vi "example.vi"() -> ()   [LabVIEW 2016]
uses:
  LS-H600-TCP Client.lvclass
  C:/Program Files (x86)/National Instruments/LabVIEW 2016/vi.lib/ActorFramework/Actor/Actor.lvclass
  LS-H600-TCP Client.lvclass/LS-H600-TCP Client.ctl
  <vilib>/ActorFramework/Message Enqueuer/Message Enqueuer.lvclass/Message Enqueuer.ctl
  <vilib>/ActorFramework/Message Enqueuer/Enqueue.vi
  C:/Program Files (x86)/National Instruments/LabVIEW 2016/vi.lib/ActorFramework/Message/Message.lvclass
  <vilib>/ActorFramework/Stop Msg/Stop Msg.lvclass
  <vilib>/ActorFramework/Message Priority Queue/Priority Enqueue.vi
  <vilib>/ActorFramework/Actor/Actor.lvclass
panel:
  out "连接错误":errorcluster
  out "数据输出":string
  out "data":T1
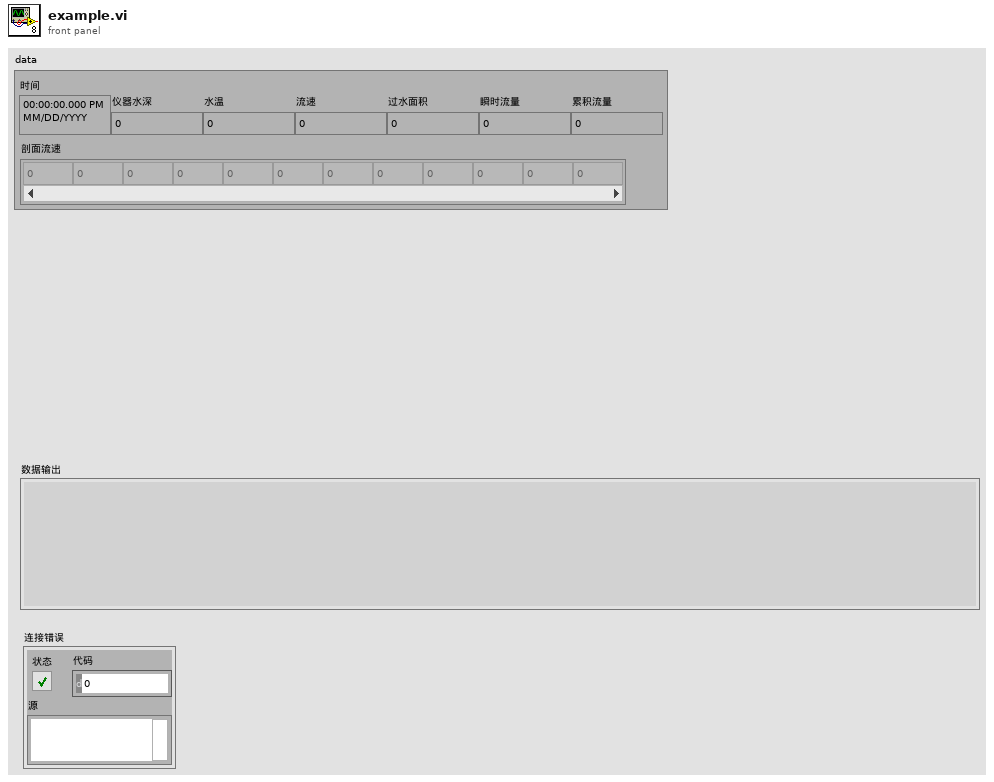
[diagram p1: front panel]
types:
  T1 = cluster{"时间":timestamp, "仪器水深":dbl, "水温":dbl, "流速":dbl, "过水面积":dbl, "瞬时流量":dbl, "累积流量":dbl, "剖面流速":dbl[]}
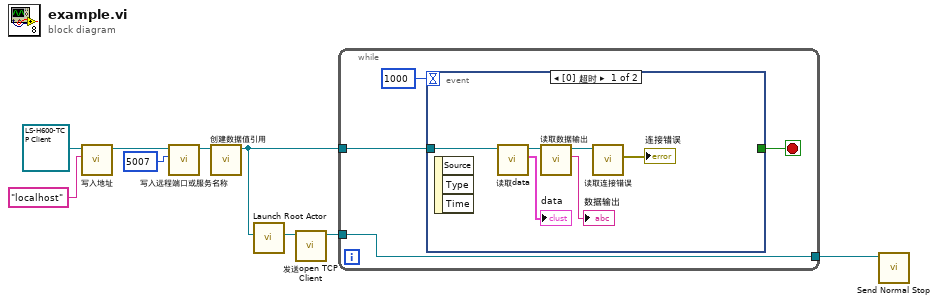
[diagram p0: block diagram]
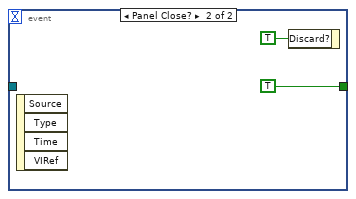
[diagram p2: hidden frame]
diagram:
  n1 = call "写入地址.vi"("地址"="localhost", "LS-H600-TCP Client输入"=refnum<class "LS-H600-TCP Client.lvclass"> refnum ("LS-H600-TCP Client.lvlib:LS-H600-TCP Client.lvclass")) -> ("LS-H600-TCP Client输出"=w8:refnum<class "LS-H600-TCP Client.lvclass">)  [unwired: 8 in, 1 out]
  n2 = call "写入远程端口或服务名称.vi"("远程端口或服务名称"=u16 5007, "LS-H600-TCP Client输入"=w8) -> ("LS-H600-TCP Client输出"=w3:refnum<class "LS-H600-TCP Client.lvclass">)  [unwired: 8 in, 1 out]
  n3 = call "创建数据值引用.vi"("LS-H600-TCP Client 输入"=w3) -> ("LS-H600-TCP Client 输出"=w2:refnum<class "LS-H600-TCP Client.lvclass">)  [unwired: 9 in, 1 out]
  n4 = call <vilib>:"Launch Root Actor.vi"("Actor"=w2) -> ("Actor's Enqueuer"=w5:refnum<class "Message Enqueuer.lvclass">)  [unwired: 9 in, 1 out]
  n5 = call "发送open TCP Client.vi"("Message Enqueuer"=w5) -> ("Message Enqueuer out"=w4:refnum<class "Message Enqueuer.lvclass">)  [unwired: 9 in, 1 out]
  n6 = while {
    tunnel: w4 -> [w12]
    tunnel: w2 -> [w13]
    tunnel: [w12] -> w1
    stop <- w10 stop-if-true
    n7 = event shown="[0] 超时" {
      selector: _ -> [_ _]
      dyn-events: _ -> [_ _]
      timeout: 1000 -> [_ _]
      tunnel: w13 -> [w18 _]
      tunnel: [_ TRUE] -> w10
      event Timeout {
        n8 = event-data() -> ()  [unwired: 1 in, 3 out]
        n9 = call "读取data.vi"("LS-H600-TCP Client输入"=w18) -> ("data"=→"data":T1, "LS-H600-TCP Client输出"=w17:refnum<class "LS-H600-TCP Client.lvclass">)  [unwired: 8 in, 1 out]
        n10 = call "读取数据输出.vi"("LS-H600-TCP Client输入"=w17) -> ("数据输出"=→"数据输出":string, "LS-H600-TCP Client输出"=w15:refnum<class "LS-H600-TCP Client.lvclass">)  [unwired: 8 in, 1 out]
        n11 = call "读取连接错误.vi"("LS-H600-TCP Client输入"=w15) -> ("连接错误"=→"连接错误":errorcluster)  [unwired: 8 in, 2 out]
      }
      event Panel Close? {
        n12 = event-data() -> ()  [unwired: 1 in, 4 out]
        n13 = event-data("Discard?"=TRUE ("放弃？")) -> ()  [unwired: 1 in, 1 out]
      }
    }
  }
  n14 = call <vilib>:"Send Normal Stop.vi"("Message Enqueuer"=w1) -> ()  [unwired: 10 in, 1 out]
